vi "Circle_Area_Poly.vi"   [LabVIEW 2011]
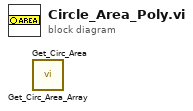
[diagram p0: block diagram]
diagram:
  n1 = call "Get_Circ_Area_Array.vi"() -> ()  [unwired: 5 in, 1 out]
  n2 = call "Get_Circ_Area.vi"() -> ()  [unwired: 5 in, 1 out]
